vi "Compute HSL Color Ranges.vi"(8 "Margins":cluster{"Hue":i32, "Sat":i32, "Lum":i32}, 9 "Luminance":i32, 10 "Saturation":i32, 11 "Hue":i32) -> (1 "Lum Range":cluster{i32, i32}, 2 "Sat Range":cluster{i32, i32}, 3 "Hue Range":cluster{i32, i32})   [LabVIEW 2013]
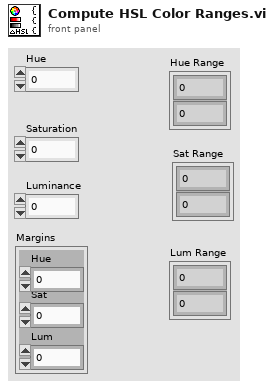
[diagram p1: front panel]
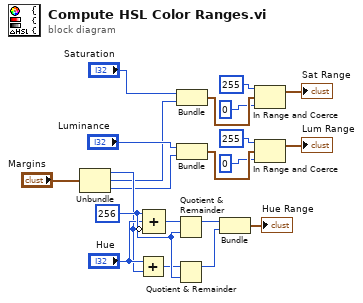
[diagram p0: block diagram]
diagram:
  w21 = 256
  n1 = Unbundle("Margins") -> ("Hue"=w14:i32, "Sat"=w5:i32, "Lum"=w11:i32)
  n2 = Add(x="Hue", y=w14) -> (x+y=w18:i32)
  n3 = Compound Arithmetic op=ADD(w21, "Hue", invert w14) -> (w19:i32)
  n4 = Quotient & Remainder(x=w19, y=w21) -> (x-y*floor(x/y)=w17:i32)  [unwired: 1 out]
  n5 = Quotient & Remainder(x=w18, y=w21) -> (x-y*floor(x/y)=w16:i32)  [unwired: 1 out]
  n6 = Bundle("Saturation"="Saturation", "Sat"=w5) -> (w4:cluster{"Saturation":i32, "Sat":i32})  [unwired: 1 in]
  n7 = Bundle("Luminance"="Luminance", "Lum"=w11) -> (w10:cluster{"Luminance":i32, "Lum":i32})  [unwired: 1 in]
  n8 = Bundle(w17, w16) -> (→"Hue Range":cluster{i32, i32})  [unwired: 1 in]
  n9 = In Range and Coerce(upper limit=255, x=w4, lower limit=0) -> (coerced(x)=→"Sat Range":cluster{"Saturation":i32, "Sat":i32})  [unwired: 1 out]
  n10 = In Range and Coerce(upper limit=255, x=w10, lower limit=0) -> (coerced(x)=→"Lum Range":cluster{"Luminance":i32, "Lum":i32})  [unwired: 1 out]
